vi "Configure Pulse List Sweep.vi"(0 "VISA resource name":refnum<visa-resource-name>="USB0::0x05E6::0x2461::04090181::INSTR", 1 "Delay (0)":dbl format="%#_9g", 2 "Count (1)":i32=1, 3 "Pulse Width":dbl format="%#_9g", 4 "Pulse Off Time":dbl format="%#_9g", 5 "error in (no error)":errorcluster, 6 "Start Index":u32=1, 7 "Buffer Name (defbuffer1)":string, 8 "Source Mode  (0: Voltage)":u16(ring) items=["Voltage", "Current"], 9 "Enable Measure (True)":bool=TRUE, 11 "Fail Abort (True)":bool=TRUE) -> (14 "VISA resource name out":refnum<visa-resource-name>="USB0::0x05E6::0x2461::04090181::INSTR", 19 "error out":errorcluster={"status"=TRUE, "code"=-1074000000, "source"="Keithley 2450.lvlib:Error Query.vi<ERR>\nInstrument reports:\n1135,\"Parameter 8, Syntax error, expected valid numeric or name parameter;1;2016/01/27 22:12:30.285\"\r\n0,\"No error;0;0 0\"\r\n\n\n\n<b>Complete call chain:</b>\r\n     Keithley 2450.lvlib:Error Query.vi\r\n     Keithley 2450.lvlib:Configure Pulse List Sweep.vi"})   [LabVIEW 2018, in "Keithley 2450.lvlib"]
doc: "This command sets up a pulse sweep based on a configuration list, which allows you to customize the sweep.\n\n<B>This function is only compatible with the 2461.</B>"
uses:
  <instrlib>/Keithley 2450/Keithley 2450.lvlib
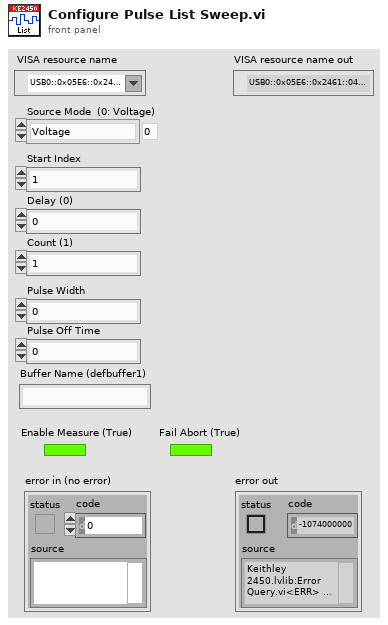
[diagram p1: front panel]
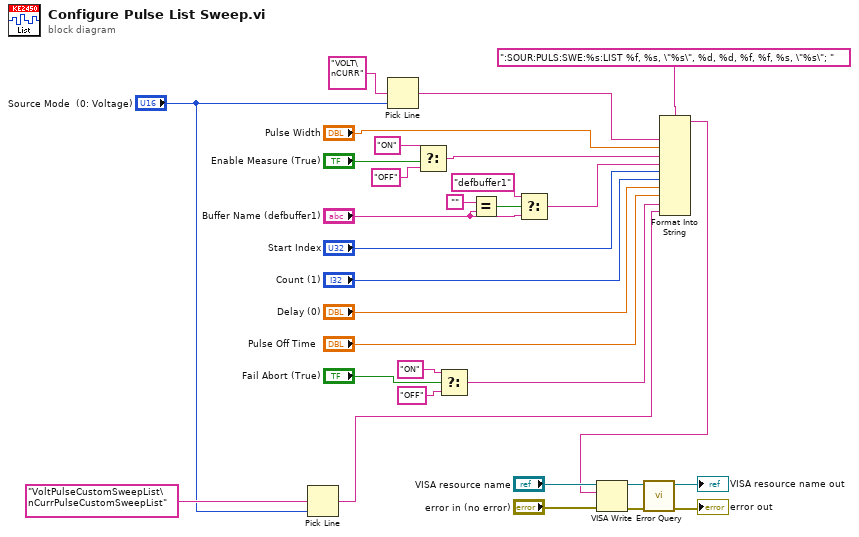
[diagram p0: block diagram]
diagram:
  n1 = Pick Line(multi-line string="VoltPulseCustomSweepList\nCurrPulseCustomSweepList" ("string (\"\")"), line index="Source Mode  (0: Voltage)") -> (output string=w3:string)  [unwired: 1 out]
  n2 = Pick Line(multi-line string="VOLT\nCURR" ("string (\"\")"), line index="Source Mode  (0: Voltage)") -> (output string=w12:string)  [unwired: 1 out]
  n3 = Select(t="ON", s="Enable Measure (True)", f="OFF") -> (s? t:f=w10:string)
  n4 = Select(t="ON" ("Buffer Name (defbuffer1)"), s="Fail Abort (True)", f="OFF" ("Buffer Name (defbuffer1)")) -> (s? t:f=w4:string)
  n5 = Equal?(x="", y="Buffer Name (defbuffer1)") -> (x = y?=w20:bool)
  n6 = Select(t="defbuffer1", s=w20, f="Buffer Name (defbuffer1)") -> (s? t:f=w9:string)
  n7 = Format Into String(format string=":SOUR:PULS:SWE:%s:LIST %f, %s, \"%s\", %d, %d, %f, %f, %s, \"%s\"; ", w12, "Pulse Width", w10, w9, "Start Index", "Count (1)", "Delay (0)", "Pulse Off Time", w4, w3) -> (resulting string=w2:string)  [unwired: 2 in, 1 out]
  n8 = VISA Write(VISA resource name="VISA resource name", write buffer=w2, error in (no error)="error in (no error)") -> (VISA resource name out=w27:refnum<visa-resource-name>, error out=w26:errorcluster)  [unwired: 1 out]
  n9 = call <instrlib>:"Error Query.vi"("error in (no error)"=w26, "VISA resource name"=w27) -> ("error out"=→"error out":errorcluster, "VISA resource name out"=→"VISA resource name out":refnum<visa-resource-name>)  [unwired: 8 out]
